vi "Check-Binary-image-storage.vi"(8 "error in":errorcluster, 10 "Analysis params. ref.":refnum<data-value>, 11 "Save?":bool) -> (0 "error IO":errorcluster, 3 "Passed?":bool)   [LabVIEW 2013, in "CameraVision.lvlib" / "CV-Storage.lvclass"]
uses:
  CV-Storage.lvclass
  Analysis/CV-Analysis.lvclass
  Analysis/CV-Analysis.lvclass/CV-Analysis.ctl
  Analysis/Read Melt-pool characteristics.vi
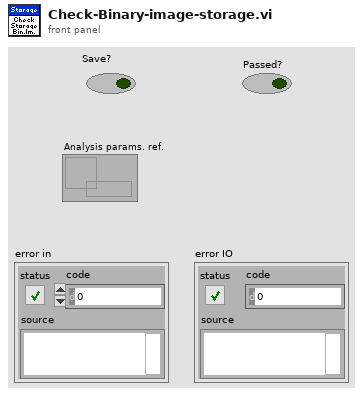
[diagram p1: front panel]
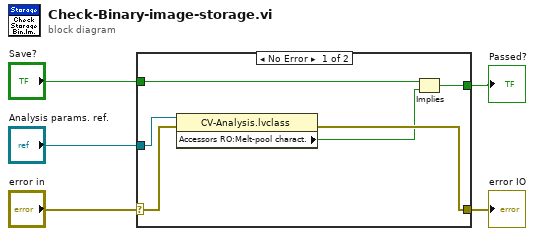
[diagram p0: block diagram]
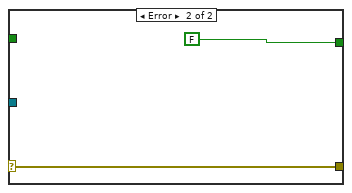
[diagram p2: hidden frame]
diagram:
  n1 = case shown="No Error" "error in" {
    selector: "error in" -> [w8 w12]
    tunnel: "Analysis params. ref." -> [w9 _]
    tunnel: [w7 w12] -> w4
    tunnel: [w11 FALSE] -> w5
    tunnel: "Save?" -> [w10 _]
    frame No Error {
      n2 = property class="CV-Analysis.lvclass"(reference=w9, error in=w8) -> (error out=w7:errorcluster, "Accessors RO:Melt-pool charact."=w6:bool)  [unwired: 1 out]
      n3 = Implies(1:w6, 2:w10) -> (0:w11:bool)
    }
    frame Error {
    }
  }
  "Passed?" <- w5
  "error IO" <- w4
